vi "close.vi"(8 "error in (no error)":errorcluster, 11 "HSDIO in":refnum<class "HSDIO.lvclass">) -> (0 "error out":errorcluster, 3 "HSDIO out":refnum<class "HSDIO.lvclass">)   [LabVIEW 2013, in "HSDIO.lvclass"]
uses:
  HSDIO.lvclass
  HSDIO.lvclass/HSDIO.ctl
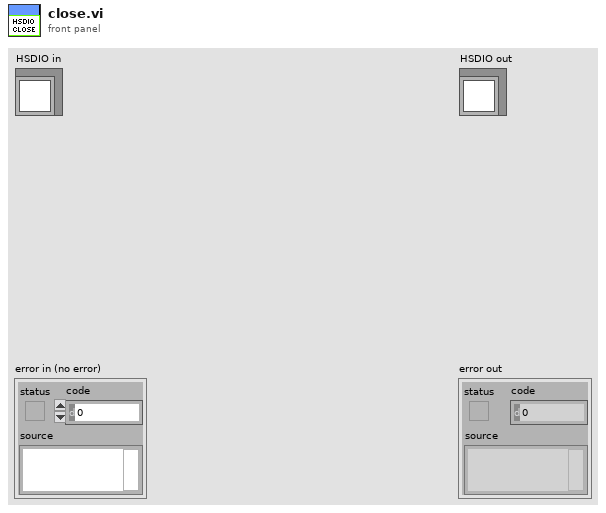
[diagram p1: front panel]
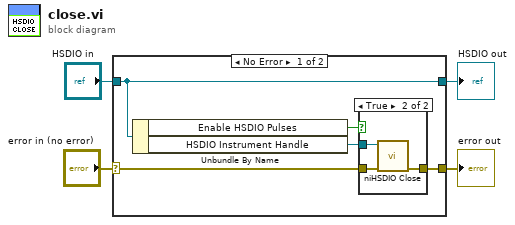
[diagram p0: block diagram]
diagram:
  n1 = case shown="No Error" "error in (no error)" {
    selector: "error in (no error)" -> [w9 w15]
    tunnel: [w8 w15] -> w3
    tunnel: [w7 w14] -> w1
    tunnel: "HSDIO in" -> [w7 w14]
    frame No Error {
      n2 = Unbundle By Name(w7) -> ("Enable HSDIO Pulses"=w5:bool, "HSDIO Instrument Handle"=w6:refnum<k15>)
      n3 = case shown="True" w5 {
        tunnel: w9 -> [w10 w13]
        tunnel: [w10 w12] -> w8
        tunnel: w6 -> [_ w11]
        frame False {
        }
        frame True {
          n4 = call <instrlib>:"niHSDIO Close.vi"("error in (no error)"=w13, "instrument handle"=w11) -> ("error out"=w12:errorcluster)  [unwired: 9 in]
        }
      }
    }
    frame Error {
    }
  }
  "error out" <- w3
  "HSDIO out" <- w1
